vi "Get Task.vi"(11 "DAQmx Base CFG in":refnum<class "DAQmx Base CFG.lvclass">) -> (2 "Task":refnum<k21>, 3 "DAQmx Base CFG out":refnum<class "DAQmx Base CFG.lvclass">)   [LabVIEW 2024, in "DAQmx Base CFG.lvclass"]
uses:
  DAQmx Base CFG.lvclass
  DAQmx Base CFG.lvclass/DAQmx Base CFG.ctl
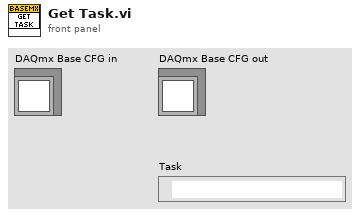
[diagram p1: front panel]
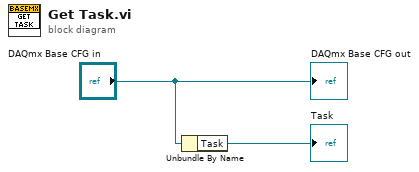
[diagram p0: block diagram]
diagram:
  n1 = Unbundle By Name("DAQmx Base CFG in") -> ("Task"=→"Task":refnum<k21>)
  "DAQmx Base CFG out" <- "DAQmx Base CFG in"
